vi "ToPythonVersionString.vi"(11 "python version":T1) -> (3 "python version string":string)   [LabVIEW 2023]
doc: "Helper VI to convert from the Python version enum to a version string that is the input to the Open Python Session node."
uses:
  PythonVersionsEnum.ctl
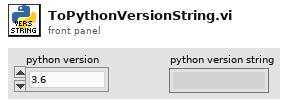
[diagram p1: front panel]
types:
  T1 = typedef "PythonVersionsEnum.ctl" = enum16{"3.6", "3.7", "3.8", "3.9", "3.10"}
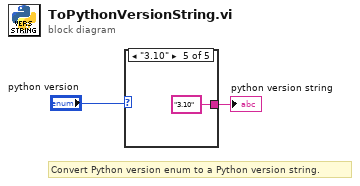
[diagram p0: block diagram]
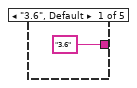
[diagram p2: hidden frame]
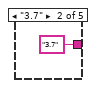
[diagram p3: hidden frame]
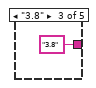
[diagram p4: hidden frame]
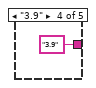
[diagram p5: hidden frame]
diagram:
  # "Convert Python version enum to a Python version string."
  n1 = case shown="\"3.10\"" "python version" {
    tunnel: ["3.6" ("python version") "3.7" ("python version") "3.8" ("python version") "3.9" ("python version") "3.10" ("python version")] -> w1
    frame "3.6", Default {
    }
    frame "3.7" {
    }
    frame "3.8" {
    }
    frame "3.9" {
    }
    frame "3.10" {
    }
  }
  "python version string" <- w1
